vi "Calibrate.vi"(8 "error in (no error)":errorcluster, 11 "AlphaStep One in":refnum<class "AlphaStep One.lvclass">) -> (0 "error out":errorcluster, 3 "AlphaStep One out":refnum<class "AlphaStep One.lvclass">)   [LabVIEW 2015, in "AlphaStep One.lvclass"]
uses:
  AlphaStep One.lvclass
  AlphaStep One.lvclass/AlphaStep One.ctl
  Serial Device/Serial Device.lvclass
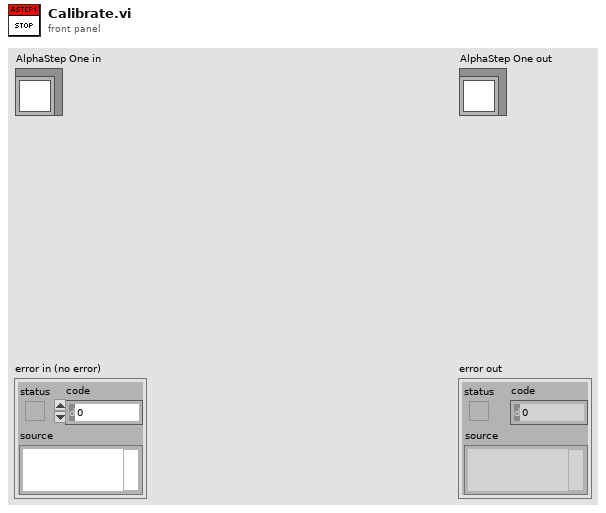
[diagram p1: front panel]
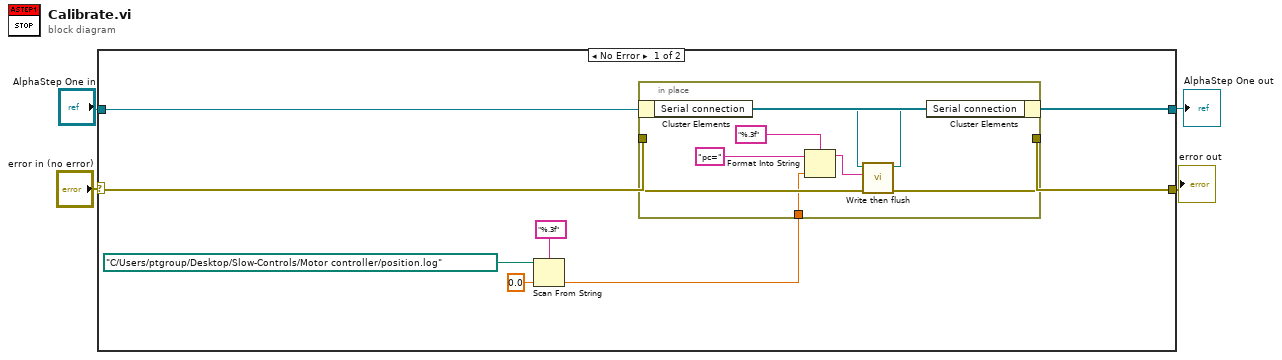
[diagram p0: block diagram]
diagram:
  n1 = case shown="No Error" "error in (no error)" {
    selector: "error in (no error)" -> [w10 w21]
    tunnel: "AlphaStep One in" -> [w12 w22]
    tunnel: [w11 w22] -> w3
    tunnel: [w9 w21] -> w2
    frame No Error {
      n2 = Scan From String("%.3f" ("format (%.3f)"), path "C:/Users/ptgroup/Desktop/Slow-Controls/Motor controller/position.log" ("Path"), default 1=0.0 ("default value 1")) -> (output 1=w5:dbl)  [unwired: 1 in, 2 out]
      n3 = in-place {
        in-place-border: w10 -> [w19]
        in-place-border: [w18] -> w9
        in-place-border: w5 -> [w13]
        n4 = in-place-cluster #1(w12) -> ("Serial connection"=w20:refnum<class "Serial Device.lvclass">)
        n5 = Format Into String(format string="%.3f" ("TX Data"), initial string="pc=", w13) -> (resulting string=w15:string)  [unwired: 1 in, 1 out]
        n6 = call "Write then flush.vi"("error in (no error)"=w19, "TX Data"=w15, "Serial Device in"=w20) -> ("error out"=w18:errorcluster, "Serial Device out"=w17:refnum<class "Serial Device.lvclass">)  [unwired: 7 in]
        n7 = in-place-cluster #1("Serial connection"=w17) -> (w11:refnum<class "AlphaStep One.lvclass">)
      }
    }
    frame Error {
    }
  }
  "error out" <- w2
  "AlphaStep One out" <- w3
